vi "Database.Handler.ReconnectAll.vi"(8 "error in (no error)":errorcluster, 11 "Data in":T1) -> (0 "error out":errorcluster, 3 "Data out":T1)   [LabVIEW 2016]
uses:
  Database.Handler.Data.ctl
  Database.Handler.Data.Status.ctl
  Database.Handler.Data.Sets.ctl
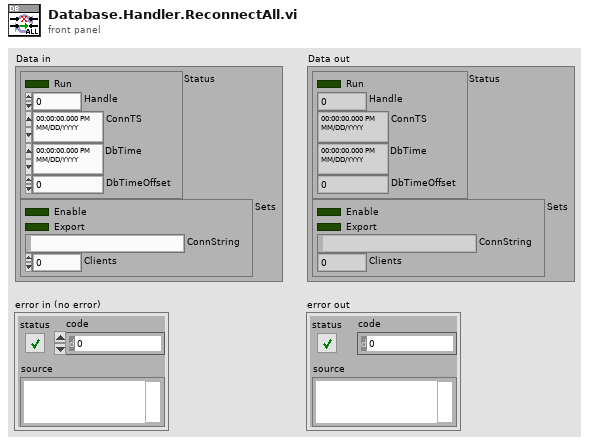
[diagram p1: front panel]
types:
  T1 = typedef "Database.Handler.Data.ctl" = cluster{"Status":T2, "Sets":T3}
  T2 = typedef "Database.Handler.Data.Status.ctl" = cluster{"Run":bool, "Handle":i32, "ConnTS":timestamp, "DbTime":timestamp, "DbTimeOffset":dbl}
  T3 = typedef "Database.Handler.Data.Sets.ctl" = cluster{"Enable":bool, "Export":bool, "ConnString":string, "Clients":i32}
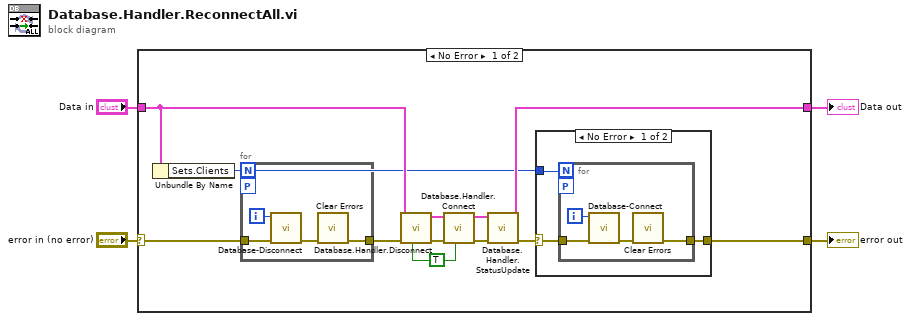
[diagram p0: block diagram]
diagram:
  n1 = case shown="No Error" "error in (no error)" {
    selector: "error in (no error)" -> [w10 w30]
    tunnel: [w7 w29] -> w4
    tunnel: "Data in" -> [w16 w29]
    tunnel: [w15 w30] -> w2
    frame No Error {
      w13 = TRUE ("ReInitDLL (F)")
      n2 = Unbundle By Name(w16) -> ("Sets.Clients"=w5:i32)
      n3 = for {
        N: w5 -> [_]
        tunnel: w10 -> [w28]
        tunnel: [w25] -> w11
        workers-P: _ -> [_]
        i -> [w26]
        n4 = call "Database-Disconnect.vi"("error in"=w28, "Idx"=w26) -> ("error out"=w27:errorcluster)  [unwired: 9 in]
        n5 = call <vilib>:"Clear Errors.vi"("error in (no error)"=w27) -> ("error out"=w25:errorcluster)  [unwired: 5 in, 1 out]
      }
      n6 = call "Database.Handler.Disconnect.vi"("ReInitDLL (F)"=w13, "error in (no error)"=w11, "Data in"=w16) -> ("error out"=w12:errorcluster, "Data out"=w14:T1)  [unwired: 7 in]
      n7 = call "Database.Handler.Connect.vi"("ReInitDLL (F)"=w13, "error in"=w12, "Data in"=w14) -> ("error out"=w9:errorcluster, "Data out"=w8:T1)  [unwired: 7 in]
      n8 = call "Database.Handler.StatusUpdate.vi"("error in (no error)"=w9, "Data in"=w8) -> ("error out"=w6:errorcluster, "Data out"=w7:T1)  [unwired: 8 in]
      n9 = case shown="No Error" w6 {
        selector: w6 -> [w18 w24]
        tunnel: w5 -> [w17 _]
        tunnel: [w19 w24] -> w15
        frame No Error {
          n10 = for {
            N: w17 -> [_]
            tunnel: w18 -> [w23]
            tunnel: [w20] -> w19
            workers-P: _ -> [_]
            i -> [w21]
            n11 = call "Database-Connect.vi"("error in"=w23, "Idx"=w21) -> ("error out"=w22:errorcluster)  [unwired: 9 in]
            n12 = call <vilib>:"Clear Errors.vi"("error in (no error)"=w22) -> ("error out"=w20:errorcluster)  [unwired: 5 in, 1 out]
          }
        }
        frame Error {
        }
      }
    }
    frame Error {
    }
  }
  "Data out" <- w4
  "error out" <- w2
